vi "Read from device.vi"() -> (2 "Humidity":dbl, 3 "temperature":dbl)   [LabVIEW 2016]
uses:
  RDingUSB.dll
panel:
  out "error out":errorcluster
  in  "Specify location":string
  out "Read work?":bool
  out "Write work?":bool
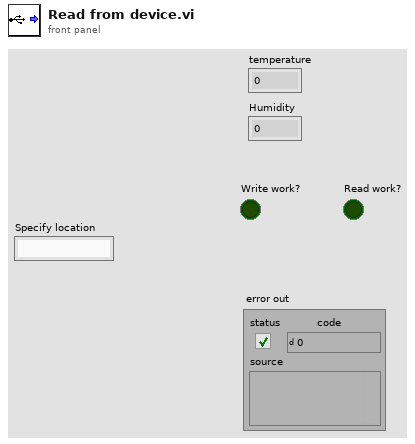
[diagram p1: front panel]
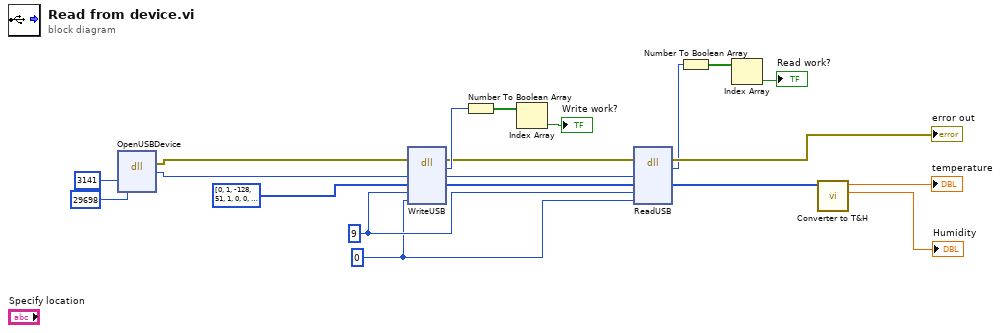
[diagram p0: block diagram]
diagram:
  w4 = u64 0 ("number0fBytesWrite")
  w6 = 9 ("bytesCount")
  n1 = dll-call lib="C:/Users/patrick/Documents/GitHub/TEMPerHUM/TEMPerHUM via DLL/RDingUSB.dll" fn="OpenUSBDevice"("VID"=3141, "PID"=29698) -> (error out=w17:errorcluster, "return type"=w18:i64)  [unwired: 5 in, 1 out]
  n2 = dll-call lib="C:/Users/patrick/Documents/GitHub/TEMPerHUM/TEMPerHUM via DLL/RDingUSB.dll" fn="WriteUSB"(error in=w17, "deviceHandle"=w18, "buffer"=i8[] [0, 1, -128, 51, 1, 0, 0, 0, 0] ("Array"), "bytesCount"=w6, "number0fBytesWrite"=w4) -> (error out=w2:errorcluster, "return type"=w9:i32, "deviceHandle"=w7:i64, "buffer"=w5:i8[])  [unwired: 4 in, 1 out]
  n3 = Number To Boolean Array(number=w9) -> (Boolean array=w10:bool[])
  n4 = Index Array(array=w10) -> (element=→"Write work?":bool)  [unwired: 1 in]
  n5 = dll-call lib="C:/Users/patrick/Documents/GitHub/TEMPerHUM/TEMPerHUM via DLL/RDingUSB.dll" fn="ReadUSB"(error in=w2, "deviceHandle"=w7, "buffer"=w5, "bytesCount"=w6, "number0fBytesRead"=w4) -> (error out=→"error out":errorcluster, "return type"=w14:i32, "buffer"=w15:u8[])  [unwired: 5 in, 1 out]
  n6 = Number To Boolean Array(number=w14) -> (Boolean array=w13:bool[])
  n7 = Index Array(array=w13) -> (element=→"Read work?":bool)  [unwired: 1 in]
  n8 = call "Converter to T&H.vi"("buffer"=w15) -> ("Humidity"=→"Humidity":dbl, "Temperature"=→"temperature":dbl)  [unwired: 9 in]
